vi "Test Process Config File as Directory Path.vi"(8 "error in (no error)":errorcluster, 11 "Process Test In":refnum<class "Process Test.lvclass">) -> (0 "error out":errorcluster, 3 "Process Test Out":refnum<class "Process Test.lvclass">)   [LabVIEW 2020, in "Process Test.lvclass"]
uses:
  Process Test.lvclass
  C:/Program Files (x86)/National Instruments/LabVIEW 2020/vi.lib/Asteme/LUnit/Test Case.lvclass
  Framework/Process/Process.lvclass
  Framework/Process/Process.lvclass/Process.ctl
  <vilib>/Asteme/LUnit/Test Case.lvclass/Test Case.ctl
  <vilib>/Asteme/LUnit/LUnit Assertion Result.lvclass/LUnit Assertion Result.ctl
  Framework/Process/Public/Get Lifecycle State.vi
  Framework/Process/Private/SubVIs/Wait for finish.vi
  Framework/Process/Protected/Messaging/Enqueue Message.vi
  Framework/Process/Private/SubVIs/Set Lifecycle State.vi
  <vilib>/Asteme/LUnit/Palette/Fail.vi
  <vilib>/Asteme/LUnit/Palette/Pass.vi
  <vilib>/Asteme/LUnit/Set Assertion Type.vi
  <vilib>/Utility/error.llb/Clear Errors.vi
  <vilib>/Asteme/LUnit/Add test result.vi
  <vilib>/Asteme/LUnit/LUnit Write Passed.vi
  <vilib>/Asteme/LUnit/LUnit Get Test Case.vi
  <vilib>/Asteme/LUnit/LUnit Write Message.vi
  <vilib>/Asteme/LUnit/LUnit Write Description.vi
  <vilib>/Asteme/LUnit/LUnit Write Assertion Type.vi
  <vilib>/Asteme/LUnit/Read Test Case Name.vi
  <vilib>/Utility/error.llb/Error Cluster From Error Code.vi
  <vilib>/Asteme/LUnit/Assertion Result/LUnit Get Test Name.vi
  <vilib>/Asteme/LUnit/LUnit Assertion Result.lvclass
  <vilib>/Asteme/LUnit/Test Case.lvclass
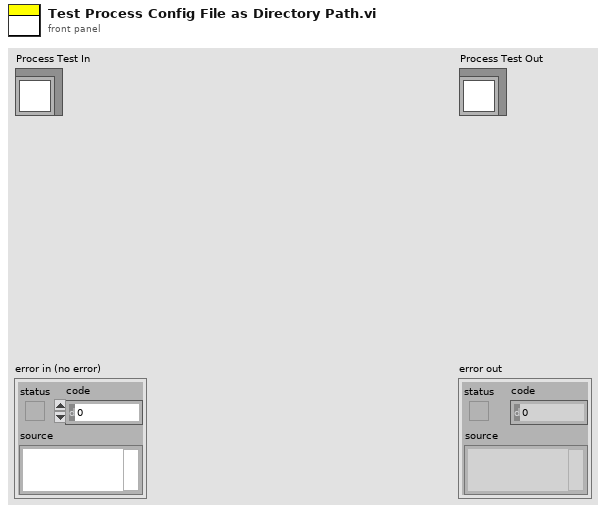
[diagram p1: front panel]
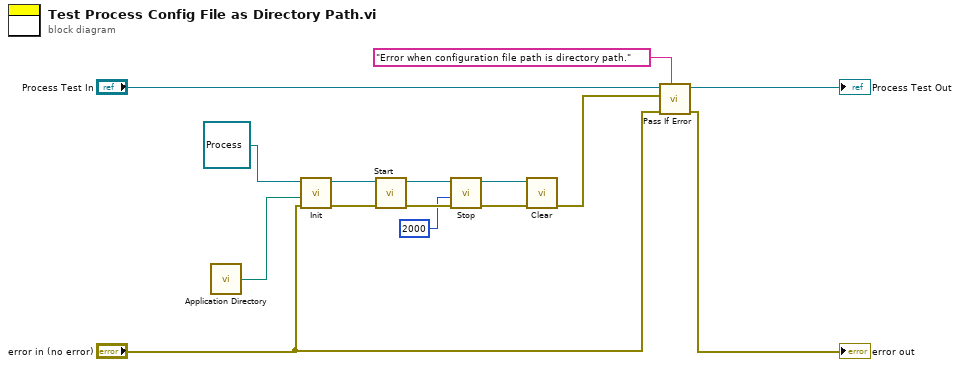
[diagram p0: block diagram]
diagram:
  n1 = call <vilib>:"Application Directory.vi"() -> ("Application Directory"=w11:path)
  n2 = call-dynamic "Init.vi"("error in (no error)"="error in (no error)", "Config File Path"=w11, "Process In"=refnum<class "Process.lvclass"> refnum ("Application.lvclass")) -> ("error out"=w12:errorcluster, "Process Out"=w14:refnum<class "Process.lvclass">)  [unwired: 7 in]
  n3 = call "Start.vi"("error in (no error)"=w12, "Process In"=w14) -> ("error out"=w3:errorcluster, "Process Out"=w13:refnum<class "Process.lvclass">)  [unwired: 8 in]
  n4 = call "Stop.vi"("error in (no error)"=w3, "timeout in ms (-1)"=2000, "Process In"=w13) -> ("error out"=w2:errorcluster, "Process Out"=w4:refnum<class "Process.lvclass">)  [unwired: 6 in, 1 out]
  n5 = call-dynamic "Clear.vi"("error in (no error)"=w2, "Process In"=w4) -> ("error out"=w9:errorcluster)  [unwired: 8 in, 1 out]
  n6 = call <vilib>:"Pass If Error.vi"("Description"="Error when configuration file path is directory path.", "error in (no error)"="error in (no error)", "Assert error"=w9, "Test Case In"="Process Test In") -> ("error out"=→"error out":errorcluster, "Test Case Out"=→"Process Test Out":refnum<class "Process Test.lvclass">)  [unwired: 6 in]
